vi "generateTemporaryFilePath.vi"(8 "error in (no error)":errorcluster, 11 "npoiDocument in":refnum<class "npoiDocument.lvclass">) -> (0 "error out":errorcluster, 2 "Unique Temporary File Path":path, 3 "npoiDocument out":refnum<class "npoiDocument.lvclass">)   [LabVIEW 2017, in "NPOI_Document.lvlib" / "npoiDocument.lvclass"]
uses:
  npoiDocument.lvclass
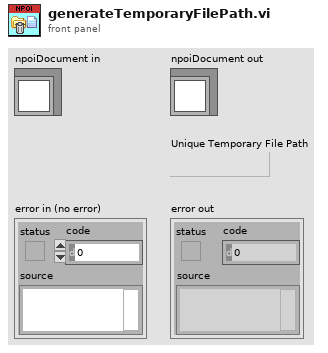
[diagram p1: front panel]
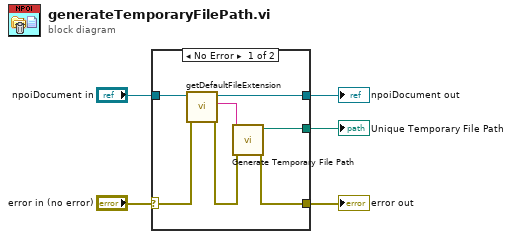
[diagram p0: block diagram]
diagram:
  n1 = case shown="No Error" "error in (no error)" {
    selector: "error in (no error)" -> [w9 w14]
    tunnel: [w11 w14] -> w4
    tunnel: [w10 w13] -> w2
    tunnel: "npoiDocument in" -> [w12 w13]
    tunnel: [w6 _] -> w1
    frame No Error {
      n2 = call-dynamic "getDefaultFileExtension.vi"("error in (no error)"=w9, "npoiDocument in"=w12) -> ("error out"=w8:errorcluster, "Default File Extension"=w7:string, "npoiDocument out"=w10:refnum<class "npoiDocument.lvclass">)  [unwired: 7 in]
      n3 = call <vilib>:"Generate Temporary File Path.vi"("error in (no error)"=w8, "Temporary File Extension (tmp)"=w7) -> ("error out"=w11:errorcluster, "Unique Temporary File Path"=w6:path)  [unwired: 8 in]
    }
    frame Error {
    }
  }
  "error out" <- w4
  "npoiDocument out" <- w2
  "Unique Temporary File Path" <- w1
